vi "Kamila_Kupidura_IB1_Projekt_OI.vi"() -> ()   [LabVIEW 2010]
uses:
  <vilib>/Analysis/8numeric.llb/1D Numeric Integration.vi
  <vilib>/Analysis/NI_AALPro.lvlib
panel:
  out "?":picture
  in  "Zapisz do .tex TXT":bool
  out "całkowice zużyta woda":dbl(slide) scale=0.0..70.0
  out "Przepływ wody w ogrodzie":dbl(graph)
  out "ilość wody":i32
  out "ilość minut":i32
  out "godziny":i32
  out "minuty":i32
  in  "opóźnienie czasowe":dbl=1.0 caption="Delay Time (s)"
  in  "?":dbl(knob) scale=0.0..19.0
  in  "basen":bool
  out "zbiorczy koncowy":dbl(slide) scale=0.0..70.0
  in  "sztuczny wodospad":bool
  out "sztuczny wodospad":dbl(slide) scale=0.0..50.0
  in  "zraszanie trawy":bool
  out "zrasznie trawy":dbl(slide) scale=0.0..50.0
  in  "kaskada":bool
  out "kaskada":dbl(slide) scale=0.0..20.0
  in  "oczko wodne":bool
  out "oczko wodne":dbl(slide) scale=0.0..50.0
  out "basen":dbl(slide) scale=0.0..50.0
  in  "włącz fontanne":bool
  out "fontanna":dbl(slide) scale=0.0..50.0
  in  "stop":bool
  in  "główny zawór":dbl(knob) scale=0.0..70.0
  out "zawór główny":dbl(slide) scale=0.0..70.0
  # "Projekt ogródka"
  # "całkowite zużycie wody"
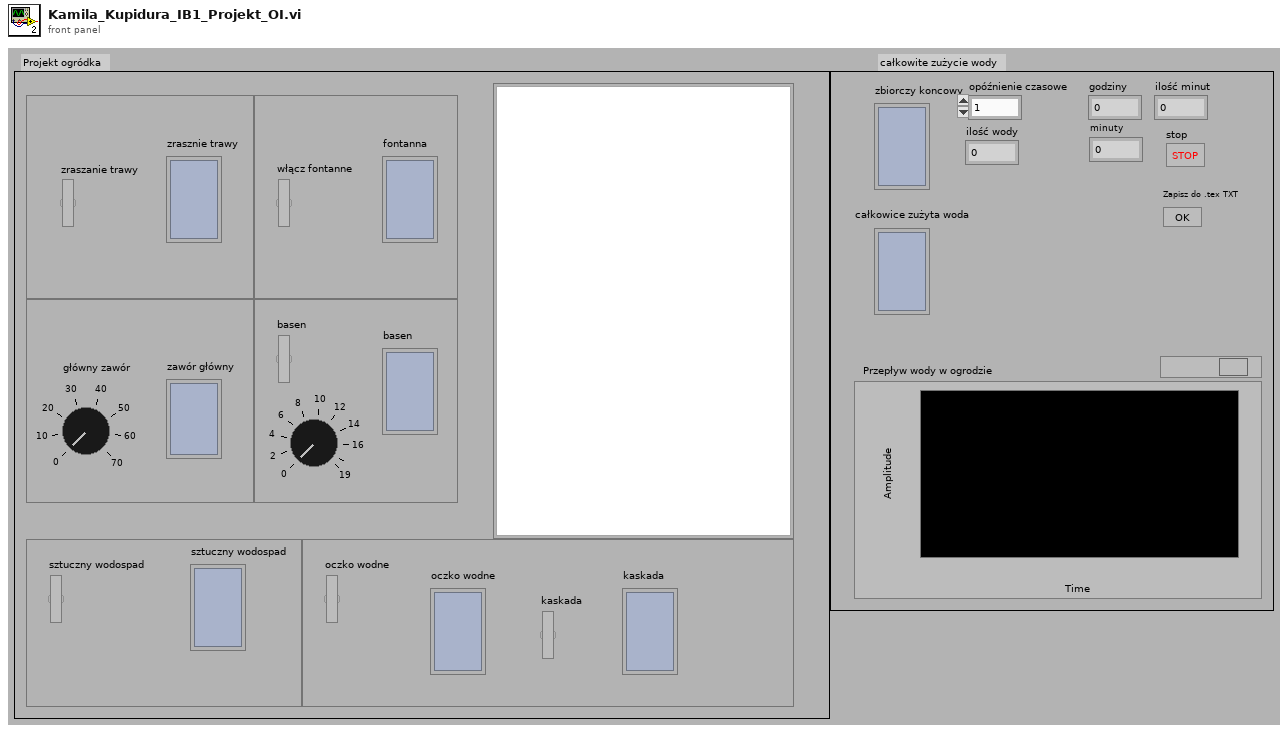
[diagram p1: front panel]
types:
  T1 = typedef "imagedata.ctl" = cluster{"image type":i32, "image depth":i32, "image":u8[], "mask":u8[], "colors":u32[], "Rectangle":cluster{"left":i16, "top":i16, "right":i16, "bottom":i16}}
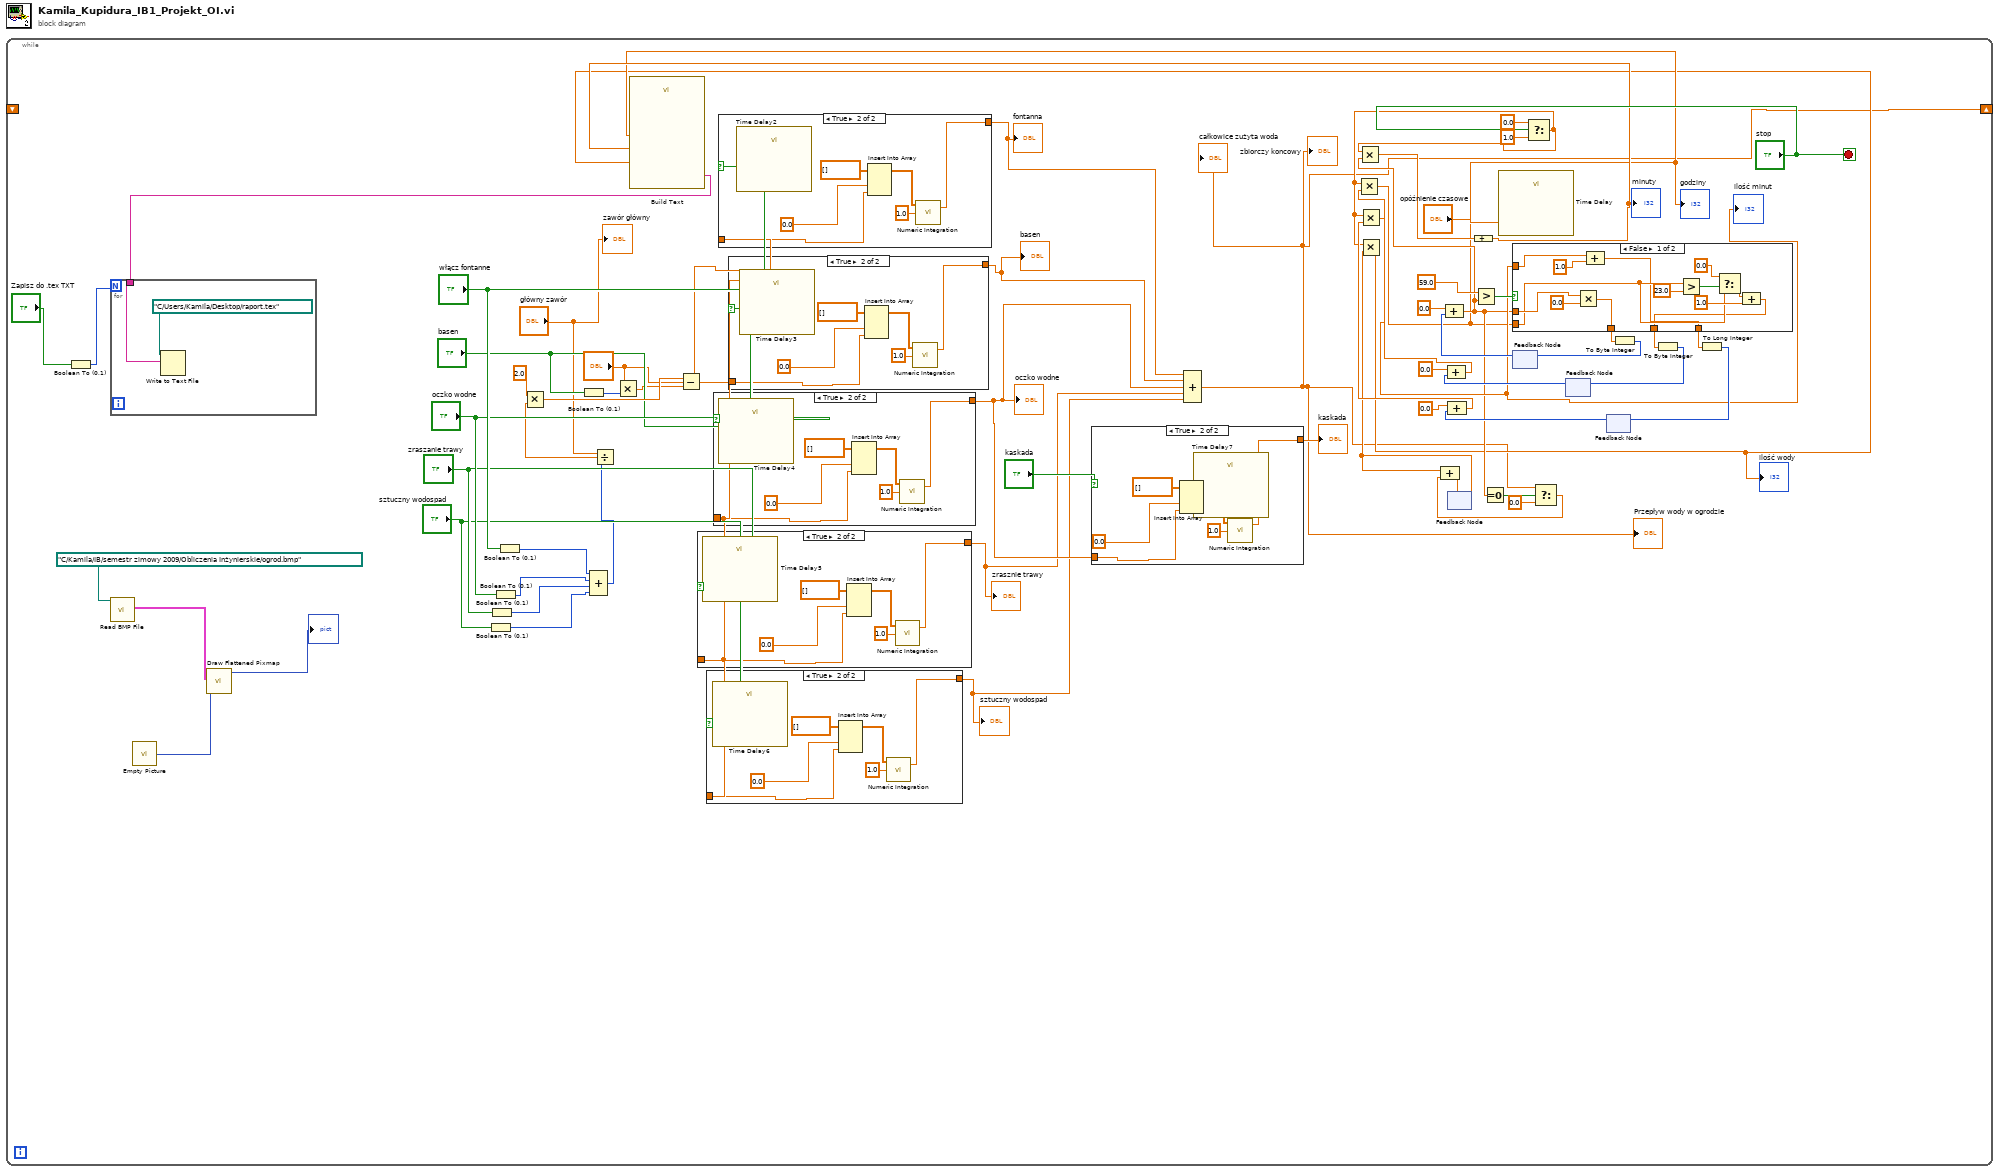
[diagram p0: block diagram]
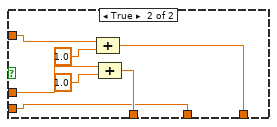
[diagram p2: hidden frame]
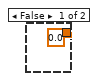
[diagram p3: hidden frame]
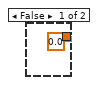
[diagram p4: hidden frame]
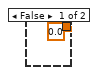
[diagram p5: hidden frame]
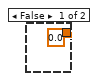
[diagram p6: hidden frame]
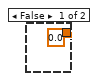
[diagram p7: hidden frame]
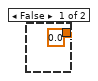
[diagram p8: hidden frame]
diagram:
  n1 = while {
    shift-right: [w5] -> _
    shift-left: _ -> [_]
    stop <- "stop" stop-if-true
    n2 = Boolean To (0,1)(Boolean="Zapisz do .tex TXT") -> (0, 1=w10:i16)
    n3 = call <vilib>:"Read BMP File.vi"("path to BMP file"=path "C:/Kamila/IB/semestr zimowy 2009/Obliczenia Inżynierskie/ogrod.bmp") -> ("image data"=w3:T1)  [unwired: 8 in, 2 out]
    n4 = call "Empty Picture"() -> ("empty picture"=w1:picture)
    n5 = call <vilib>:"Draw Flattened Pixmap.vi"("image data"=w3, "picture"=w1) -> ("new picture"=→"?":picture)  [unwired: 7 in]
    n6 = Boolean To (0,1)(Boolean="sztuczny wodospad") -> (0, 1=w50:i16)
    n7 = Boolean To (0,1)(Boolean="zraszanie trawy") -> (0, 1=w51:i16)
    n8 = Boolean To (0,1)(Boolean="oczko wodne") -> (0, 1=w52:i16)
    n9 = Boolean To (0,1)(Boolean="włącz fontanne") -> (0, 1=w53:i16)
    n10 = Boolean To (0,1)(Boolean="basen") -> (0, 1=w55:i16)
    n11 = Compound Arithmetic op=ADD(w53, w52, w51, w50) -> (w49:i16)
    n12 = Divide(x="główny zawór", y=w49) -> (x/y=w58:dbl)
    n13 = Multiply(x=2.0 ("dt"), y=w58) -> (x*y=w57:dbl)
    n14 = Multiply(x="?", y=w55) -> (x*y=w54:dbl)
    n15 = Subtract(x=w57, y=w54) -> (x-y=w19:dbl)
    n16 = case shown="True" "zraszanie trawy" {
      tunnel: w19 -> [_ w99]
      tunnel: [0.0 ("dt") w96] -> w14
      frame False {
      }
      frame True {
        n17 = call "Time Delay5"() -> ()  [unwired: 11 in, 1 out]
        n18 = Insert Into Array(array=dbl[] [], new element #1=0.0 ("dt"), new element #2=w99) -> (w98:dbl[])  [unwired: 1 in]
        n19 = call-poly <vilib>:"Numeric Integration.vi"("dt"=1.0, "Input Array"=w98) -> ("result"=w96:dbl)  [unwired: 1 in, 1 out]
      }
    }
    "zrasznie trawy" <- w14
    n20 = case shown="True" "sztuczny wodospad" {
      tunnel: w19 -> [_ w92]
      tunnel: [0.0 ("dt") w89] -> w13
      frame False {
      }
      frame True {
        n21 = call "Time Delay6"() -> ()  [unwired: 11 in, 1 out]
        n22 = Insert Into Array(array=dbl[] [], new element #1=0.0 ("dt"), new element #2=w92) -> (w91:dbl[])  [unwired: 1 in]
        n23 = call-poly <vilib>:"Numeric Integration.vi"("dt"=1.0, "Input Array"=w91) -> ("result"=w89:dbl)  [unwired: 1 in, 1 out]
      }
    }
    "sztuczny wodospad" <- w13
    n24 = case shown="True" "oczko wodne" {
      tunnel: w19 -> [_ w113]
      tunnel: [0.0 ("dt") w110] -> w15
      frame False {
      }
      frame True {
        n25 = call "Time Delay4"() -> ()  [unwired: 11 in, 1 out]
        n26 = Insert Into Array(array=dbl[] [], new element #1=0.0 ("dt"), new element #2=w113) -> (w112:dbl[])  [unwired: 1 in]
        n27 = call-poly <vilib>:"Numeric Integration.vi"("dt"=1.0, "Input Array"=w112) -> ("result"=w110:dbl)  [unwired: 1 in, 1 out]
      }
    }
    "oczko wodne" <- w15
    n28 = case shown="True" "włącz fontanne" {
      tunnel: w19 -> [_ w127]
      tunnel: [0.0 ("dt") w124] -> w17
      frame False {
      }
      frame True {
        n29 = call "Time Delay2"() -> ()  [unwired: 11 in, 1 out]
        n30 = Insert Into Array(array=dbl[] [], new element #1=0.0 ("dt"), new element #2=w127) -> (w126:dbl[])  [unwired: 1 in]
        n31 = call-poly <vilib>:"Numeric Integration.vi"("dt"=1.0, "Input Array"=w126) -> ("result"=w124:dbl)  [unwired: 1 in, 1 out]
      }
    }
    "fontanna" <- w17
    n32 = case shown="True" "basen" {
      tunnel: "?" -> [_ w120]
      tunnel: [0.0 ("dt") w117] -> w16
      frame False {
      }
      frame True {
        n33 = call "Time Delay3"() -> ()  [unwired: 11 in, 1 out]
        n34 = Insert Into Array(array=dbl[] [], new element #1=0.0 ("dt"), new element #2=w120) -> (w119:dbl[])  [unwired: 1 in]
        n35 = call-poly <vilib>:"Numeric Integration.vi"("dt"=1.0, "Input Array"=w119) -> ("result"=w117:dbl)  [unwired: 1 in, 1 out]
      }
    }
    "basen" <- w16
    n36 = case shown="True" "kaskada" {
      tunnel: w15 -> [_ w106]
      tunnel: [0.0 ("dt") w103] -> w64
      frame False {
      }
      frame True {
        n37 = Insert Into Array(array=dbl[] [], new element #1=0.0 ("dt"), new element #2=w106) -> (w105:dbl[])  [unwired: 1 in]
        n38 = call "Time Delay7"() -> ()  [unwired: 11 in, 1 out]
        n39 = call-poly <vilib>:"Numeric Integration.vi"("dt"=1.0, "Input Array"=w105) -> ("result"=w103:dbl)  [unwired: 1 in, 1 out]
      }
    }
    "kaskada" <- w64
    n40 = Compound Arithmetic op=ADD(w17, w16, w15, w14, w13) -> (w5:dbl)
    "zbiorczy koncowy" <- w5
    "Przepływ wody w ogrodzie" <- w5
    "całkowice zużyta woda" <- w5
    n41 = feedback #1() -> (w21:dbl)  [unwired: 1 in]
    n42 = call "Time Delay"("Delay Time (s)"="opóźnienie czasowe") -> ()  [unwired: 10 in, 1 out]
    n43 = feedback #2() -> (w44:i8)  [unwired: 1 in]
    n44 = Compound Arithmetic op=unknown(0.0 ("y"), w44) -> (w25:dbl)
    n45 = Greater?(x=59.0, y=w25) -> (0:w47:bool)
    n46 = Equal To 0?(x=w25) -> (x = 0?=w26:bool)
    n47 = Select(t=0.0, s="stop", f=1.0) -> (s? t:f=w20:dbl)
    n48 = Multiply(x=w20, y=w25) -> (x*y=w30:dbl)
    n49 = Multiply(x=w20, y=w21) -> (x*y=w6:dbl)
    "ilość wody" <- w6
    n50 = Compound Arithmetic op=ADD(w30) -> (w9:dbl)
    "minuty" <- w9
    n51 = Select(t=w5, s=w26, f=0.0) -> (s? t:f=w23:dbl)
    n52 = Compound Arithmetic op=ADD(w21, w23) -> (w22:dbl)
    n53 = feedback-in #1(w22) -> ()
    n54 = feedback #3() -> (w39:i8)  [unwired: 1 in]
    n55 = Compound Arithmetic op=unknown(0.0 ("y"), w39) -> (w29:dbl)
    n56 = Multiply(x=w20, y=w29) -> (x*y=w8:dbl)
    "godziny" <- w8
    n57 = call "Build Text"("h"=w8, "min"=w9, "zuzycie"=w6) -> ("Result"=w7:string)  [unwired: 11 in, 1 out]
    n58 = for {
      N: w10 -> [_]
      tunnel: w7 -> [w66]
      n59 = Write to Text File(file (use dialog)=path "C:/Users/Kamila/Desktop/raport.tex", text=w66) -> ()  [unwired: 2 in, 3 out]
    }
    n60 = feedback #4() -> (w34:i32)  [unwired: 1 in]
    n61 = Compound Arithmetic op=unknown(0.0 ("y"), w34) -> (w28:dbl)
    n62 = Multiply(x=w20, y=w28) -> (x*y=w27:dbl)
    "ilość minut" <- w27
    n63 = case shown="False" w47 {
      tunnel: [w78 w86] -> w43
      tunnel: w25 -> [w79 w85]
      tunnel: w8 -> [w72 w84]
      tunnel: [w68 w84] -> w38
      tunnel: w27 -> [w71 w83]
      tunnel: [w69 w82] -> w36
      frame False {
        n64 = Multiply(x=w79, y=0.0) -> (x*y=w78:dbl)
        n65 = Compound Arithmetic op=ADD(w71, 1.0 ("y")) -> (w69:dbl)
        n66 = Greater?(x=w72, y=23.0) -> (0:w75:bool)
        n67 = Select(t=0.0, s=w75, f=w72) -> (s? t:f=w76:dbl)
        n68 = Compound Arithmetic op=ADD(w76, 1.0 ("y")) -> (w68:dbl)
      }
      frame True {
        n69 = Compound Arithmetic op=ADD(w83, 1.0 ("y")) -> (w82:dbl)
        n70 = Compound Arithmetic op=ADD(w85, 1.0 ("y")) -> (w86:dbl)
      }
    }
    n71 = To Byte Integer(number=w43) -> (8bit integer=w42:i8)
    n72 = feedback-in #2(w42) -> ()
    n73 = To Byte Integer(number=w38) -> (8bit integer=w40:i8)
    n74 = feedback-in #3(w40) -> ()
    n75 = To Long Integer(number=w36) -> (32bit integer=w35:i32)
    n76 = feedback-in #4(w35) -> ()
    "zawór główny" <- "główny zawór"
  }
